vi "FastControl_TriggerTimeAlarm.vi"(6 "TimeToChange":u32, 7 "ResetAlarm":bool, 9 "Enable":bool, 11 "Signal":bool) -> (3 "Alarm":bool)   [LabVIEW 2019]
doc: "If <b>Enable</b> is True and <b>Signal</b> didn`t changed to True during specified time (<b>TimeToChange</b>) then <b>Alarm</b> is locked in True."
uses:
  <instrlib>/_niInstr/Basic Elements/v1/FPGA/Private/Count Up U32.vi
  <instrlib>/_niInstr/Basic Elements/v1/FPGA/niInstr Basic Elements v1 FPGA.lvlib
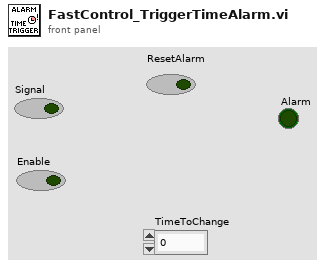
[diagram p1: front panel]
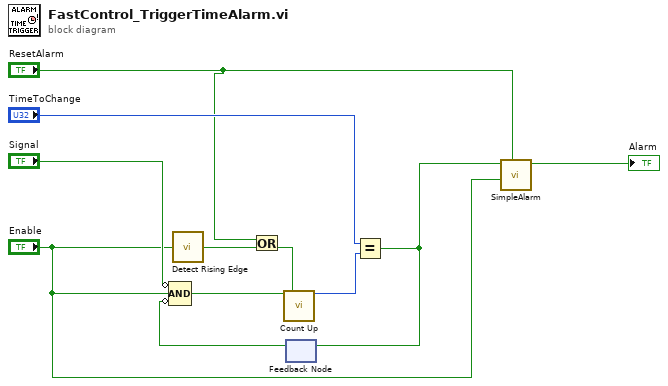
[diagram p0: block diagram]
diagram:
  n1 = call <instrlib>:"Detect Rising Edge.vi"("signal"="Enable") -> ("edge detected"=w11:bool)  [unwired: 14 in]
  n2 = Or(x="ResetAlarm", y=w11) -> (x .or. y?=w2:bool)
  n3 = feedback #1() -> (w4:bool)  [unwired: 1 in]
  n4 = Compound Arithmetic op=AND(invert "Signal", "Enable", invert w4) -> (w7:bool)
  n5 = call-poly <instrlib>:"Count Up.vi"("increment"=w7, "reset"=w2) -> ("count out"=w9:u32)  [unwired: 13 in]
  n6 = Equal?(x="TimeToChange", y=w9) -> (x = y?=w5:bool)
  n7 = feedback-in #1(w5) -> ()
  n8 = call "SimpleAlarm.vi"("ResetAlarm"="ResetAlarm", "Enable"="Enable", "AlarmCondition"=w5) -> ("Alarm"=→"Alarm":bool)  [unwired: 8 in]
